vi "Append File to Report.vi"(0 "report in":refnum<class "NI_Word.lvclass">, 1 "MS Office parameters":T1, 7 "file path":path, 9 "is spreadsheet file?(Excel)":bool, 11 "error in (no error)":errorcluster) -> (4 "report out":refnum<class "NI_Word.lvclass">, 8 "start out (Word)":i32, 10 "end out (Word)":i32, 15 "error out":errorcluster)   [LabVIEW 2023, in "NI_Word.lvclass"]
doc: "Appends the text from a text file into the current report."
uses:
  NI_Word.lvclass
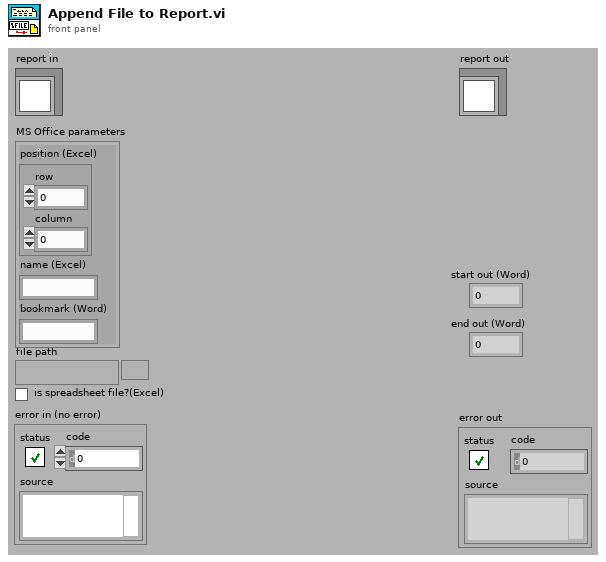
[diagram p1: front panel]
types:
  T1 = cluster{"position (Excel)":cluster{"row":i32, "column":i32}, "name (Excel)":string, "bookmark (Word)":string}
  T2 = typedef "NI_ReportGenerationCore.lvlib/Report Data Members.ctl" = cluster{"font":T3, "from template?":bool}
  T3 = typedef "NI_ReportGenerationCore.lvlib/font.ctl" = cluster{"font name":string, "font size":dbl, "bold":u16, "italic":u16, "underline":u16, "strike through":u16, "font color":u32}
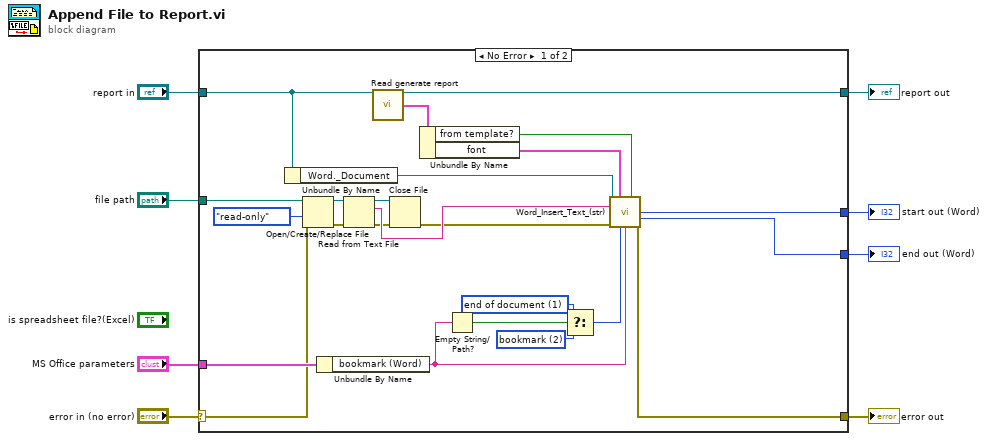
[diagram p0: block diagram]
diagram:
  n1 = case shown="No Error" "error in (no error)" {
    selector: "error in (no error)" -> [w17 w34]
    tunnel: [w16 w34] -> w7
    tunnel: [w12 w33] -> w5
    tunnel: "report in" -> [w13 w33]
    tunnel: "MS Office parameters" -> [w19 _]
    tunnel: "file path" -> [w18 _]
    tunnel: [w15 _] -> w2
    tunnel: [w14 _] -> w1
    frame No Error {
      w20 = u16 2 items=["begining of document", "end of document", "bookmark", "custom"] ("Insertion point")
      w21 = u16 1 items=["begining of document", "end of document", "bookmark", "custom"] ("Insertion point")
      n2 = Unbundle By Name(w13) -> ("Word._Document"=w25:refnum<k7>)
      n3 = Open/Create/Replace File(file path (use dialog)=w18, error in=w17, access (0:read/write)=enum16{"read/write", "read-only", "write-only"}."read-only") -> (refnum out=w28:refnum<file>, error out=w29:errorcluster)  [unwired: 4 out]
      n4 = Unbundle By Name(w19) -> ("bookmark (Word)"=w23:string)
      n5 = Read from Text File(file (use dialog)=w28, error in=w29) -> (refnum out=w27:refnum<file>, text=w32:string, error out=w26:errorcluster)  [unwired: 3 out]
      n6 = call-dynamic "Read generate report.vi"("report in"=w13) -> ("report out"=w12:refnum<class "NI_Word.lvclass">, "generate report"=w11:T2)  [unwired: 12 in, 1 out]
      n7 = Close File(refnum=w27, error in=w26) -> (error out=w31:errorcluster)  [unwired: 1 out]
      n8 = Unbundle By Name(w11) -> ("from template?"=w10:bool, "font"=w9:T3)
      n9 = Empty String/Path?(string/path=w23) -> (empty?=w22:bool)
      n10 = Select(t=w21, s=w22, f=w20) -> (s? t:f=w24:u16)
      n11 = call <vilib>:"Word_Insert_Text_(str).vi"("Word._Document"=w25, "font"=w9, "from template?"=w10, "Text"=w32, "Error in (no error)"=w31, "Insertion point"=w24, "Bookmark name"=w23) -> ("Start out"=w15:i32, "End out"=w14:i32, "Error out"=w16:errorcluster)  [unwired: 3 in, 3 out]
    }
    frame Error {
    }
  }
  "error out" <- w7
  "report out" <- w5
  "start out (Word)" <- w2
  "end out (Word)" <- w1
